vi "Measure Data 2D to Table Format.vi"(7 "Data String Format":string="%#.3p", 8 "error in":errorcluster, 10 "Y-axis Data Array Refs":refnum<vi>[](array[refnum]), 11 "X-axis Data Array Ref":refnum<vi>) -> (0 "error out":errorcluster, 2 "2D Data":string[][](array[string]), 3 "Titles":string[](array[string]))   [LabVIEW 2023]
doc: "Use this VI to convert 1D X and Y data arrays into a table format and titles using array references."
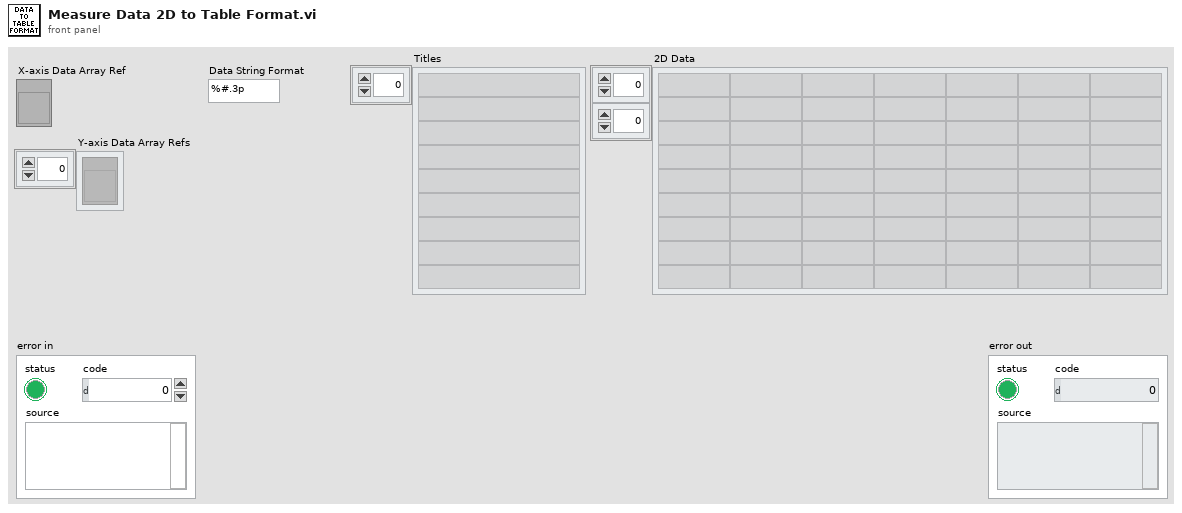
[diagram p1: front panel]
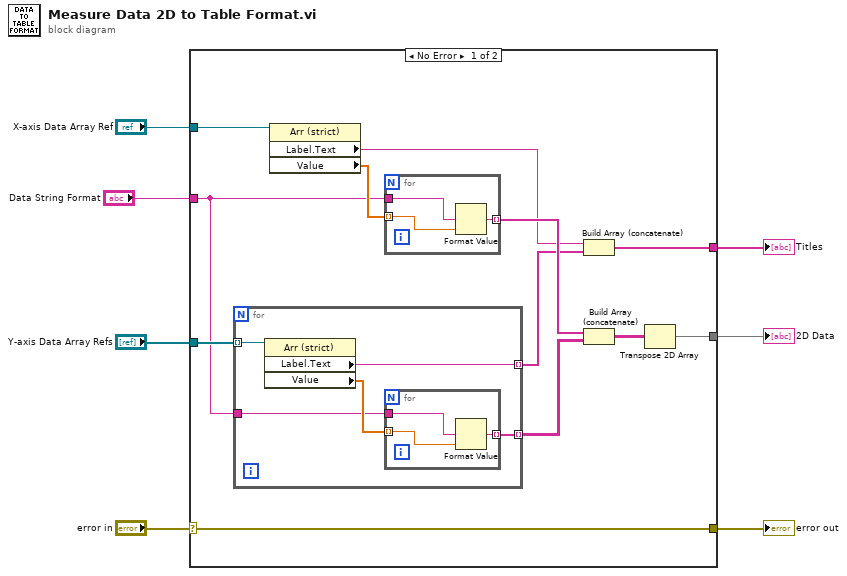
[diagram p0: block diagram]
diagram:
  n1 = case shown="No Error" "error in" {
    selector: "error in" -> [w10 w31]
    tunnel: "X-axis Data Array Ref" -> [w14 _]
    tunnel: "Y-axis Data Array Refs" -> [w13 _]
    tunnel: [w12 _] -> w5
    tunnel: [w8 _] -> w4
    tunnel: [w10 w31] -> w2
    tunnel: "Data String Format" -> [w9 _]
    frame No Error {
      n2 = for {
        tunnel: w13 -> [w27] mode=indexing
        tunnel: [w26] -> w16 mode=indexing
        tunnel: [w24] -> w17 mode=indexing
        tunnel: w9 -> [w23]
        n3 = property class="Arr (strict)"(reference=w27) -> ("Label.Text"=w26:string, "Value"=w25:dbl[])  [unwired: 1 in, 2 out]
        n4 = for {
          tunnel: [w30] -> w24 mode=indexing
          tunnel: w25 -> [w29] mode=indexing
          tunnel: w23 -> [w28]
          n5 = Format Value(format string=w28, value (0)=w29) -> (output string=w30:string)  [unwired: 1 in]
        }
      }
      n6 = property class="Arr (strict)"(reference=w14) -> ("Label.Text"=w15:string, "Value"=w18:dbl[])  [unwired: 1 in, 2 out]
      n7 = for {
        tunnel: [w22] -> w19 mode=indexing
        tunnel: w18 -> [w21] mode=indexing
        tunnel: w9 -> [w20]
        n8 = Format Value(format string=w20, value (0)=w21) -> (output string=w22:string)  [unwired: 1 in]
      }
      n9 = Build Array (concatenate)(w15, w16) -> (w12:string[])
      n10 = Build Array (concatenate)(w19, w17) -> (w11:string[][])
      n11 = Transpose 2D Array(2D array=w11) -> (transposed array=w8:string[][])
    }
    frame Error {
    }
  }
  "error out" <- w2
  "Titles" <- w5
  "2D Data" <- w4
